vi "Qn_Z.vi"(8 "Type":string, 11 "shape":string) -> (3 "Qn":dbl[](array[numeric]))   [LabVIEW 2015]
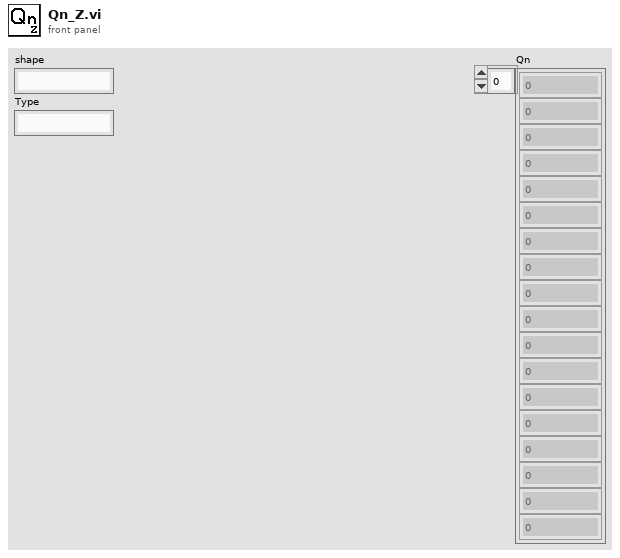
[diagram p1: front panel]
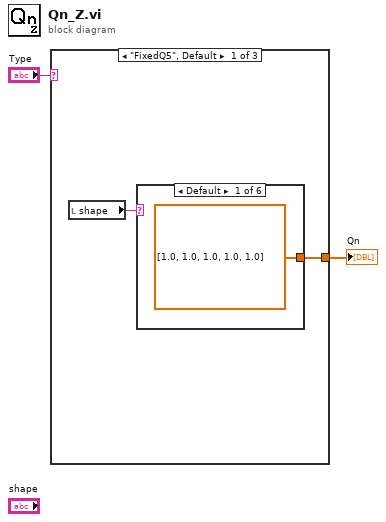
[diagram p0: block diagram]
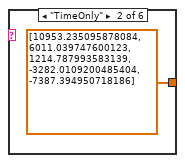
[diagram p2: hidden frame]
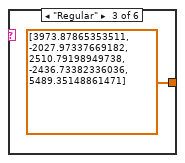
[diagram p3: hidden frame]
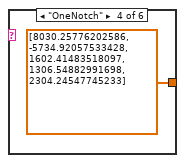
[diagram p4: hidden frame]
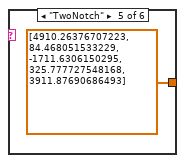
[diagram p5: hidden frame]
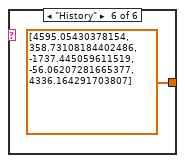
[diagram p6: hidden frame]
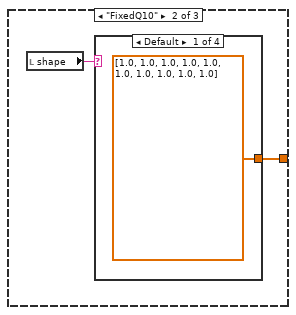
[diagram p7: hidden frame]
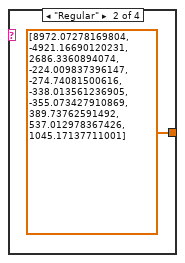
[diagram p8: hidden frame]
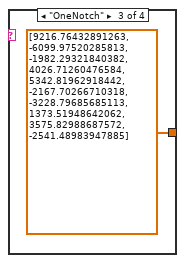
[diagram p9: hidden frame]
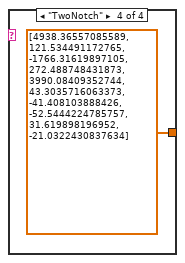
[diagram p10: hidden frame]
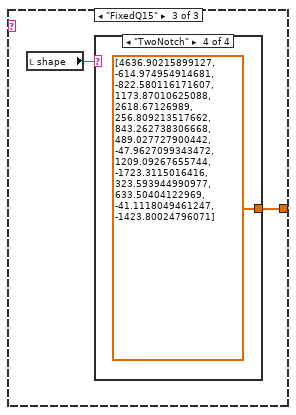
[diagram p11: hidden frame]
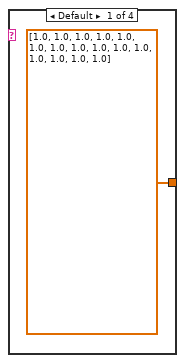
[diagram p12: hidden frame]
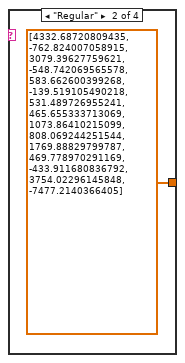
[diagram p13: hidden frame]
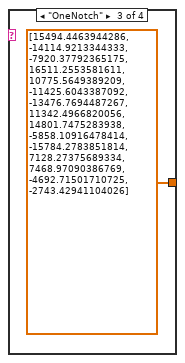
[diagram p14: hidden frame]
diagram:
  n1 = case shown="\"FixedQ5\", Default" "Type" {
    tunnel: [w3 w12 w18] -> w2
    frame "FixedQ5", Default {
      n2 = local read "shape"() -> (w4:string)
      n3 = case shown="Default" w4 {
        tunnel: [dbl[] [1.0, 1.0, 1.0, 1.0, 1.0] ("Qn") dbl[] [10953.235095878084, 6011.039747600123, 1214.787993583139, -3282.0109200485404, -7387.394950718186] ("Qn") dbl[] [3973.87865353511, -2027.97337669182, 2510.79198949738, -2436.73382336036, 5489.35148861471] ("Qn") dbl[] [8030.25776202586, -5734.92057533428, 1602.41483518097, 1306.54882991698, 2304.24547745233] ("Qn") dbl[] [4910.26376707223, 84.468051533229, -1711.6306150295, 325.777727548168, 3911.87690686493] ("Qn") dbl[] [4595.05430378154, 358.73108184402486, -1737.445059611519, -56.06207281665377, 4336.164291703807] ("Qn")] -> w3
        frame Default {
        }
        frame "TimeOnly" {
        }
        frame "Regular" {
        }
        frame "OneNotch" {
        }
        frame "TwoNotch" {
        }
        frame "History" {
        }
      }
    }
    frame "FixedQ10" {
      n4 = local read "shape"() -> (w11:string)
      n5 = case shown="Default" w11 {
        tunnel: [dbl[] [1.0, 1.0, 1.0, 1.0, 1.0, 1.0, 1.0, 1.0, 1.0, 1.0] ("Qn") dbl[] [8972.07278169804, -4921.16690120231, 2686.3360894074, -224.009837396147, -274.74081500616, -338.013561236905, -355.073427910869, 389.73762591492, 537.012978367426, 1045.17137711001] ("Qn") dbl[] [9216.76432891263, -6099.97520285813, -1982.29321840382, 4026.71260476584, 5342.81962918442, -2167.70266710318, -3228.79685685113, 1373.51948642062, 3575.82988687572, -2541.48983947885] ("Qn") dbl[] [4938.36557085589, 121.534491172765, -1766.31619897105, 272.488748431873, 3990.08409352744, 43.3035716063373, -41.408103888426, -52.5444224785757, 31.619898196952, -21.0322430837634] ("Qn")] -> w12
        frame Default {
        }
        frame "Regular" {
        }
        frame "OneNotch" {
        }
        frame "TwoNotch" {
        }
      }
    }
    frame "FixedQ15" {
      n6 = local read "shape"() -> (w17:string)
      n7 = case shown="\"TwoNotch\"" w17 {
        tunnel: [dbl[] [1.0, 1.0, 1.0, 1.0, 1.0, 1.0, 1.0, 1.0, 1.0, 1.0, 1.0, 1.0, 1.0, 1.0, 1.0] ("Qn") dbl[] [4332.68720809435, -762.824007058915, 3079.39627759621, -548.742069565578, 583.662600399268, -139.519105490218, 531.489726955241, 465.655333713069, 1073.86410215099, 808.069244251544, 1769.88829799787, 469.778970291169, -433.911680836792, 3754.02296145848, -7477.2140366405] ("Qn") dbl[] [15494.4463944286, -14114.9213344333, -7920.37792365175, 16511.2553581611, 10775.5649389209, -11425.6043387092, -13476.7694487267, 11342.4966820056, 14801.7475283938, -5858.10916478414, -15784.2783851814, 7128.27375689334, 7468.97090386769, -4692.71501710725, -2743.42941104026] ("Qn") dbl[] [4636.90215899127, -614.974954914681, -822.580116171607, 1173.87010625088, 2618.67126989, 256.809213517662, 843.262738306668, 489.027727900442, -47.9627099343472, 1209.09267655744, -1723.3115016416, 323.593944990977, 633.50404122969, -41.1118049461247, -1423.80024796071] ("Qn")] -> w18
        frame Default {
        }
        frame "Regular" {
        }
        frame "OneNotch" {
        }
        frame "TwoNotch" {
        }
      }
    }
  }
  "Qn" <- w2
